vi "UTILITY PID Correction Loop Check.vi"(8 "Error In":errorcluster, 9 "ErrorPassBand(%)":dbl, 10 "GPM Target(3)":dbl, 11 "GPM reading":dbl) -> (0 "Error Out":errorcluster, 3 "Going into Correction Loop?":bool)   [LabVIEW 2018]
panel:
  out "abs(x)":dbl
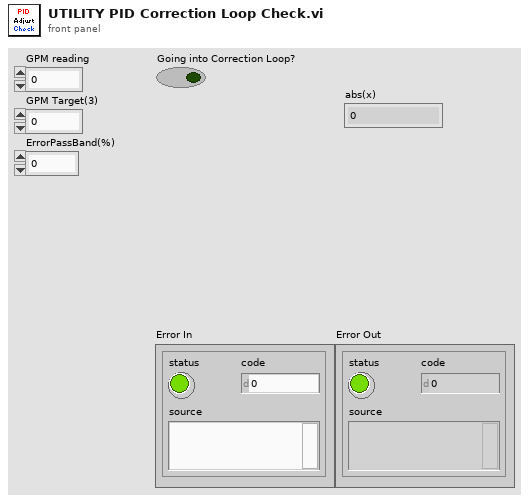
[diagram p1: front panel]
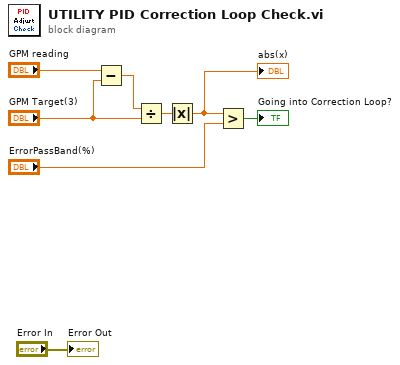
[diagram p0: block diagram]
diagram:
  n1 = Subtract(x="GPM reading", y="GPM Target(3)") -> (x-y=w5:dbl)
  n2 = Divide(x=w5, y="GPM Target(3)") -> (x/y=w2:dbl)
  n3 = Absolute Value(x=w2) -> (abs(x)=w3:dbl)
  "abs(x)" <- w3
  n4 = Greater?(x=w3, y="ErrorPassBand(%)") -> (0:→"Going into Correction Loop?":bool)
  "Error Out" <- "Error In"
